vi "Get Report Settings.vi"(0 "report in":refnum<class "NI_HTML.lvclass">, 11 "error in (no error)":errorcluster) -> (4 "report out":refnum<class "NI_HTML.lvclass">, 6 "text options":T1, 10 "font settings":T2, 14 "text color":u32(colorbox), 15 "error out":errorcluster)   [LabVIEW 2015, in "NI_HTML.lvclass"]
doc: "Retrieves information about the current font and text settings of a given report."
uses:
  <vilib>/Utility/NIReport.llb/HTML/NI_HTML.lvclass
  <vilib>/Utility/NIReport.llb/HTML/NI_HTML.lvclass/NI_HTML.ctl
  <vilib>/Utility/NIReport.llb/NI_ReportGenerationCore.lvlib
panel:
  out "color - RGB":cluster{"red":u8, "green":u8, "blue":u8}
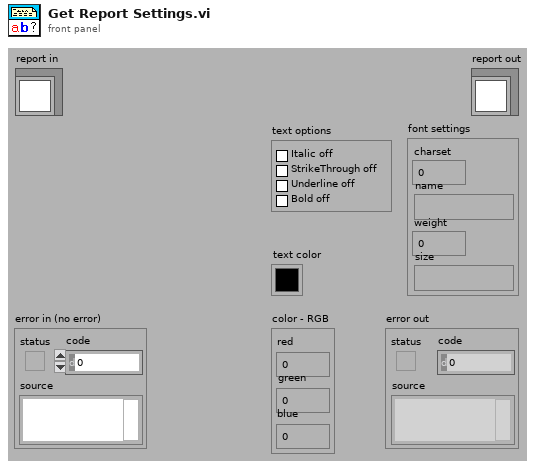
[diagram p1: front panel]
types:
  T1 = cluster{"Italic":bool, "StrikeThrough":bool, "Underline":bool, "Bold":bool}
  T2 = cluster{"charset":i16, "name":string, "weight":i16, "size":string}
  T3 = typedef "NI_ReportGenerationCore.lvlib/HTML Report Data.ctl" = cluster{"Body Text":string, "Font Tag":string, "Title Text":string, "Header Text":string, "Footer Text":string, "Image List":path[]}
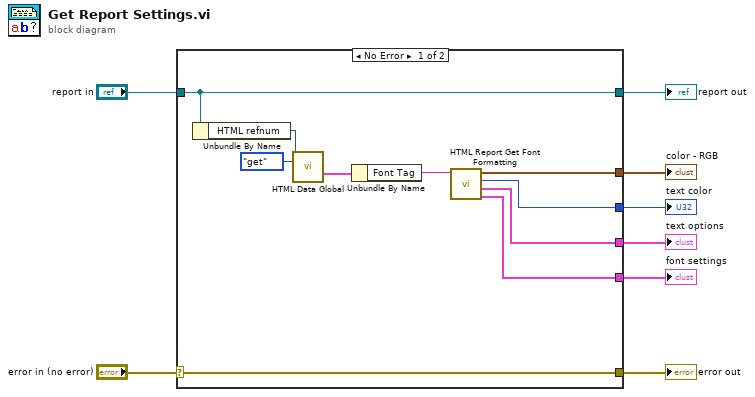
[diagram p0: block diagram]
diagram:
  n1 = case shown="No Error" "error in (no error)" {
    selector: "error in (no error)" -> [w18 w20]
    tunnel: [w18 w20] -> w7
    tunnel: [w10 w19] -> w5
    tunnel: "report in" -> [w10 w19]
    tunnel: [w17 _] -> w4
    tunnel: [w16 _] -> w3
    tunnel: [w15 _] -> w2
    tunnel: [w14 _] -> w1
    frame No Error {
      n2 = Unbundle By Name(w10) -> ("HTML refnum"=w13:u32)
      n3 = call <vilib>:"HTML Data Global.vi"("HTML refnum"=w13, "menu"=enum16{"init", "get", "set", "delete"}."get") -> ("HTML report data out"=w12:T3)  [unwired: 1 in, 12 out]
      n4 = Unbundle By Name(w12) -> ("Font Tag"=w9:string)
      n5 = call <vilib>:"HTML Report Get Font Formatting.vi"("String In"=w9) -> ("font settings"=w14:T2, "Text Options"=w15:T1, "Color Box"=w16:u32, "Output Element"=w17:cluster{"red":u8, "green":u8, "blue":u8})  [unwired: 3 out]
    }
    frame Error {
    }
  }
  "error out" <- w7
  "report out" <- w5
  "color - RGB" <- w4
  "text color" <- w3
  "text options" <- w2
  "font settings" <- w1
